vi "Configure AC Line Trigger Slope.vi"(8 "error in (no error)":errorcluster {"code" format="%.0x"}, 10 "AC Line Slope (Positive)":string(combo)="POS", 11 "VISA Resource Name":refnum<visa-resource-name>) -> (0 "error out":errorcluster {"code" format="%.0x"}, 3 "VISA Resource Name Out":refnum<visa-resource-name>)   [LabVIEW 2011, in "Agilent 546XX Series.lvlib"]
doc: "This VI configures the oscilloscope for AC Line triggering.\n\nNotes:\n\n(1) This VI affects instrument behavior only if the Trigger Type is AC Line Trigger. Call the ag546xx Configure Trigger VI to set the Trigger Type before you call this VI."
uses:
  Agilent 546XX Series.lvlib
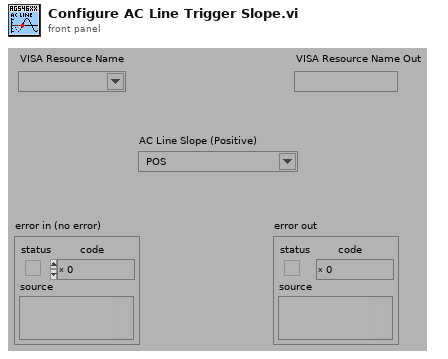
[diagram p1: front panel]
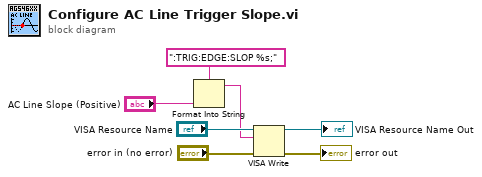
[diagram p0: block diagram]
diagram:
  n1 = Format Into String(format string=":TRIG:EDGE:SLOP %s;", "AC Line Slope (Positive)") -> (resulting string=w1:string)  [unwired: 2 in, 1 out]
  n2 = VISA Write(VISA resource name="VISA Resource Name", write buffer=w1, error in (no error)="error in (no error)") -> (VISA resource name out=→"VISA Resource Name Out":refnum<visa-resource-name>, error out=→"error out":errorcluster)  [unwired: 1 out]
